vi "Aire3.vi"() -> ()   [LabVIEW 2023]
uses:
  <vilib>/MakerHub/LINX/LMH-LINX.lvlib
  <vilib>/MakerHub/LINX/Public/Peripherals/Analog/Analog Read 1 Chan.vi
  <vilib>/MakerHub/LINX/Public/Peripherals/Digital/Digital Write 1 Chan.vi
  <vilib>/MakerHub/LINX/Public/Utilities/Open Serial.vi
panel:
  in  "stop":bool
  out "Boolean":bool
  in  "Smoke Value":dbl
  out "Smoke output":dbl(knob) scale=0.0..1025.0
  in  "Serial Port":refnum<visa-resource-name>="N/A"
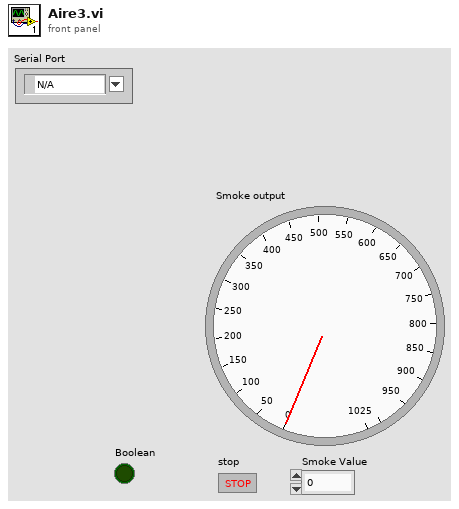
[diagram p1: front panel]
types:
  T1 = typedef "LMH-LINX.lvlib/LINX Ref.ctl" = cluster{"IO":T2, "Interface":T3, "LINX Device Config":T4}
  T2 = typedef "LMH-LINX.lvlib/Platform.ctl" = enum16{"Remote", "Local"}
  T3 = typedef "LMH-LINX.lvlib/Interface.ctl" = enum16{"Serial", "TCP"}
  T4 = typedef "LMH-LINX.lvlib/Device.lvlib/LINX Device Config.ctl" = cluster{"Interface":T3, "COM Port":refnum<visa-resource-name>, "TCP Configuration":T5, "Device Family":u8, "Device ID":u8, "Device Name":string, "TCP Ref":refnum<k5>, "Channels":T6}
  T5 = typedef "LMH-LINX.lvlib/Device.lvlib/TCP Config.ctl" = cluster{"IP Address":string, "Port":u16}
  T6 = typedef "LMH-LINX.lvlib/Channels.ctl" = cluster{"DI":u8[], "DO":u8[], "AI":u8[], "AO":u8[], "PWM":u8[], "QE":u8[], "UART":u8[], "I2C 2":u8[], "SPI":u8[], "CAN":u8[], "Servo":u8[], "AI Ref (V)":dbl, "AI Resolution (Bits)":u8, "AO Ref (V)":dbl, "AO Resolution (Bits)":u8}
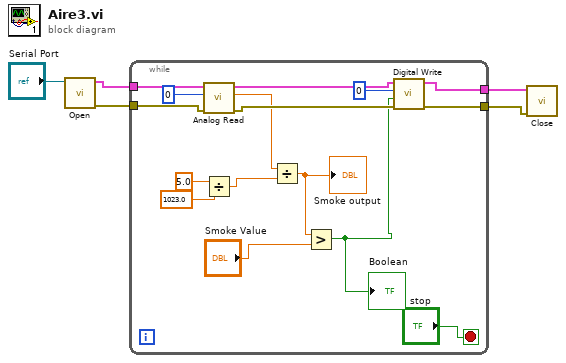
[diagram p0: block diagram]
diagram:
  n1 = call-poly <vilib>:"Open.vi"("Serial Port"="Serial Port") -> ("Error Out"=w3:errorcluster, "LINX Resource"=w2:T1)  [unwired: 8 in, 1 out]
  n2 = while {
    tunnel: [w19] -> w5
    tunnel: [w18] -> w4
    tunnel: w3 -> [w17]
    tunnel: w2 -> [w16]
    stop <- "stop" stop-if-true
    n3 = call-poly <vilib>:"Analog Read.vi"("Error In"=w17, "Analog Channel"=u8 0, "LINX Resource"=w16) -> ("Error Out"=w20:errorcluster, "Voltage"=w10:dbl, "LINX Resource"=w21:T1)  [unwired: 5 in, 1 out]
    n4 = Divide(x=5.0, y=1023.0) -> (x/y=w11:dbl)
    n5 = Divide(x=w10, y=w11) -> (x/y=w9:dbl)
    "Smoke output" <- w9
    n6 = Greater?(x=w9, y="Smoke Value") -> (0:w7:bool)
    "Boolean" <- w7
    n7 = call-poly <vilib>:"Digital Write.vi"("Error In"=w20, "Output Value"=w7, "DO Channel"=u8 0, "LINX Resource"=w21) -> ("Error Out"=w18:errorcluster, "LINX Resource"=w19:T1)  [unwired: 6 in]
  }
  n8 = call <vilib>:"Close.vi"("Error In"=w4, "LINX Resource"=w5) -> ()  [unwired: 9 in, 1 out]
